vi "LVFunction_Read reg fo haso.vi"(4 "error in (no error)":errorcluster) -> (0 "error out":errorcluster, 3 "Path to config files":path)   [LabVIEW 2020]
uses:
  <vilib>/registry/registry.llb/Registry RtKey.ctl
  <vilib>/registry/registry.llb/Registry SAM.ctl
  <vilib>/registry/registry.llb/Read Registry Value Simple STR.vi
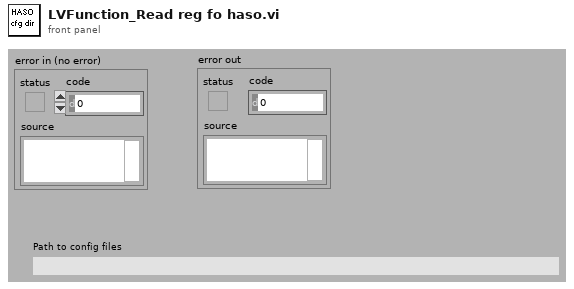
[diagram p1: front panel]
types:
  T1 = typedef "Registry SAM.ctl" = enum32{"KEY_QUERY_VALUE", "KEY_SET_VALUE", "KEY_CREATE_SUB_KEY", "KEY_ENUMERATE_SUB_KEYS", "KEY_NOTIFY", "KEY_CREATE_LINK", "KEY_READ", "KEY_WRITE", "KEY_ALL_ACCESS", "KEY_READ | KEY_WRITE"}
  T2 = typedef "Registry RtKey.ctl" = enum32{"HKEY_CLASSES_ROOT", "HKEY_CURRENT_USER", "HKEY_LOCAL_MACHINE", "HKEY_USERS", "HKEY_PERFORMANCE_DATA", "HKEY_CURRENT_CONFIG", "HKEY_DYN_DATA"}
  T3 = typedef "Registry refnum.ctl" = refnum<k1>
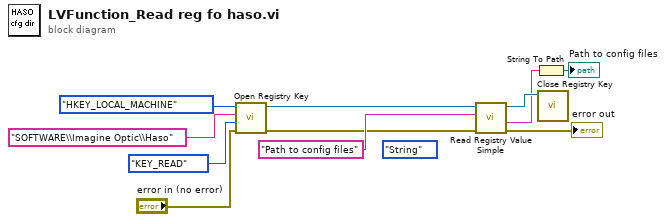
[diagram p0: block diagram]
diagram:
  (unwired) enum16{"String", "Binary", "DWORD"}."String" ("simple data type")
  n1 = call <vilib>:"Open Registry Key.vi"("error in (no error)"="error in (no error)", "security access mask (KEY_READ | KEY_WRITE)"=Registry_SAM."KEY_READ", "subkey"="SOFTWARE\\Imagine Optic\\Haso", "root key (HKEY_LOCAL_MACHINE)"=Registry_RtKey."HKEY_LOCAL_MACHINE") -> ("error out"=w7:errorcluster, "refnum out"=w6:T3)  [unwired: 6 in]
  n2 = call-poly <vilib>:"Read Registry Value Simple.vi"("error in (no error)"=w7, "value"="Path to config files", "refnum"=w6) -> ("error out"=→"error out":errorcluster, "String/Binary data"=w2:string, "refnum out"=w5:T3)  [unwired: 3 in, 1 out]
  n3 = String To Path(string=w2) -> (path=→"Path to config files":path)
  n4 = call <vilib>:"Close Registry Key.vi"("refnum"=w5) -> ()  [unwired: 6 in, 1 out]
